vi "Test Serializer API.vi"() -> ()   [LabVIEW 2015, in "Serializer.lvlib"]
doc: "Serializer API Tester."
uses:
  Serializer.lvlib
panel:
  in  "close":bool
  in  "open":bool
  in  "conf":bool
  in  "config":string="{\"Plugin\":\"MOXAIP\",\"IP\":\"192.168.20.118\",\"Port\":4001}"
  in  "Send":bool
  in  "String":string
  in  "Run as Singleton?":bool
  in  "Show Block Diagram":bool
  in  "Refresh Modules":bool
  out "Active Modules":string[](array[string])
  in  "Stop Module":bool
  in  "Select Module":i32(ring)=-1 caption="Select Module\nTo send Request to" items=["All"=-1]
  in  "Run New Module":bool
  in  "Hide Module Panel":bool
  in  "Show Module Panel":bool
  out "Status":string
  # "This VI tests the API for the Module."
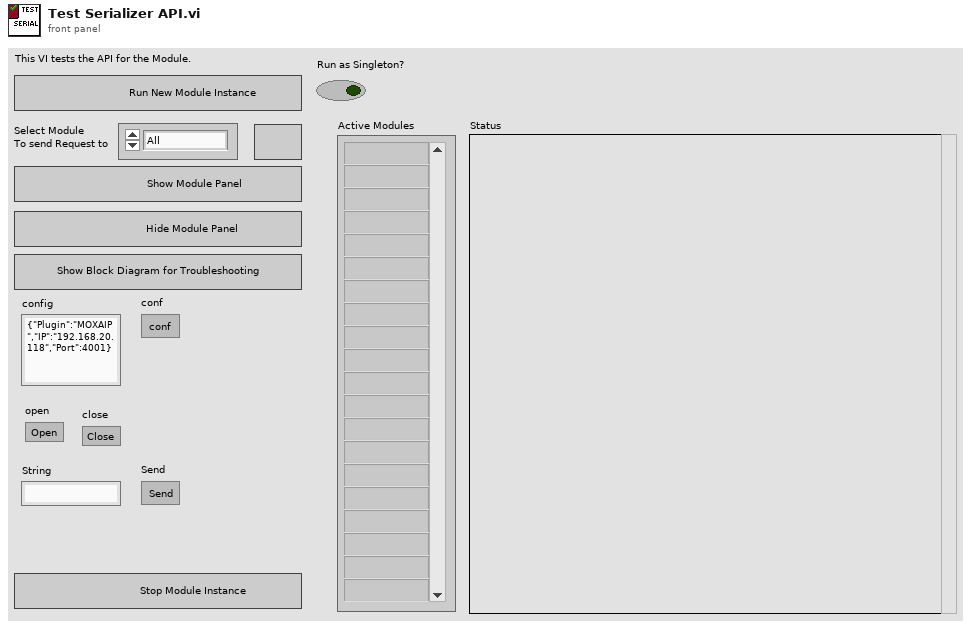
[diagram p1: front panel]
types:
  T1 = typedef "Serializer.lvlib/Broadcast Events--cluster.ctl" = cluster{"Module Did Init":refnum<user-event>, "Status Updated":refnum<user-event>, "Error Reported":refnum<user-event>, "Module Did Stop":refnum<user-event>, "Update Module Execution Status":refnum<user-event>, "Received":refnum<user-event>}
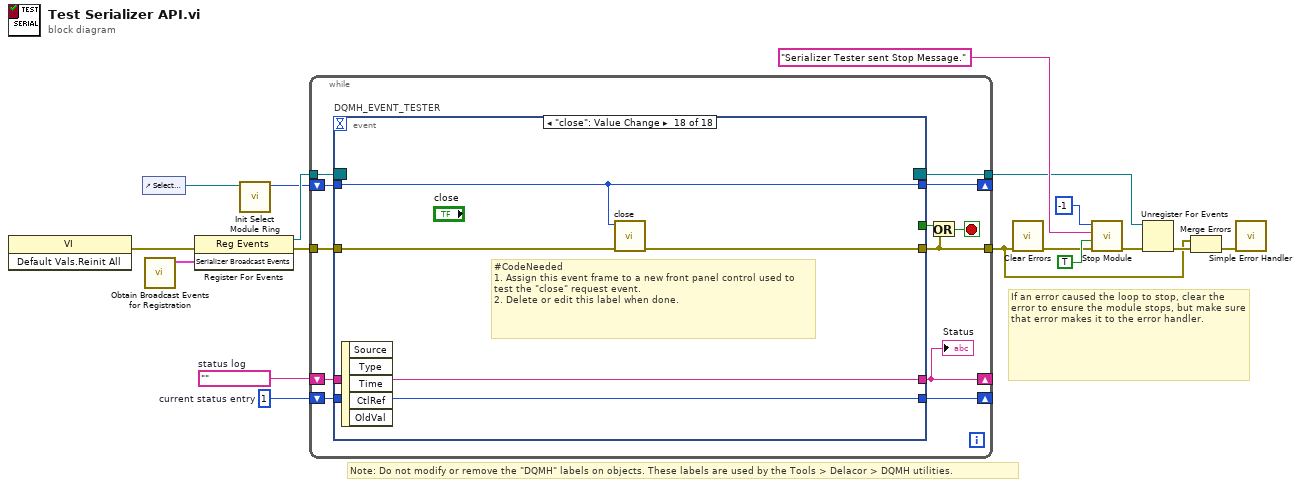
[diagram p0: block diagram]
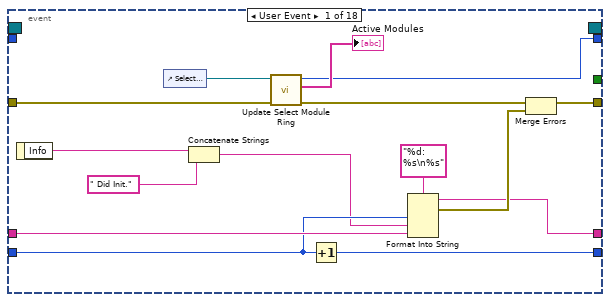
[diagram p2: hidden frame]
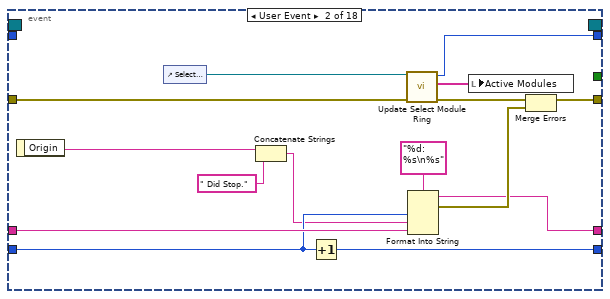
[diagram p3: hidden frame]
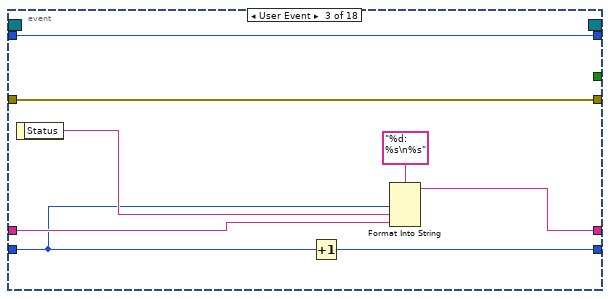
[diagram p4: hidden frame]
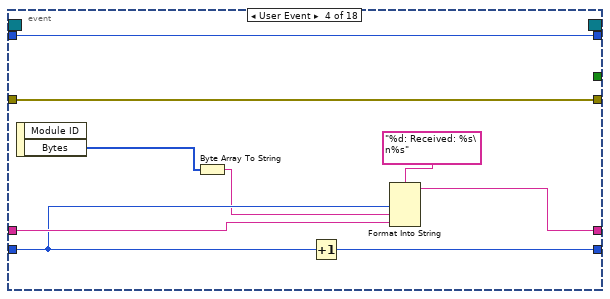
[diagram p5: hidden frame]
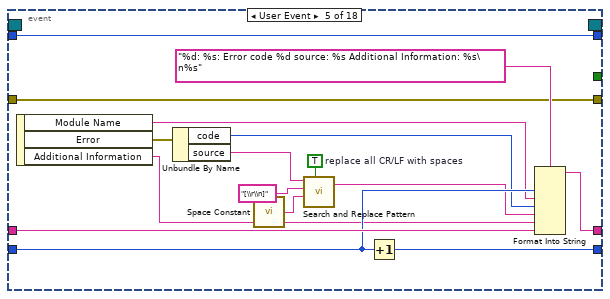
[diagram p6: hidden frame]
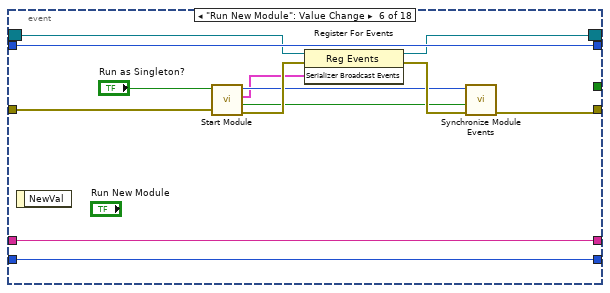
[diagram p7: hidden frame]
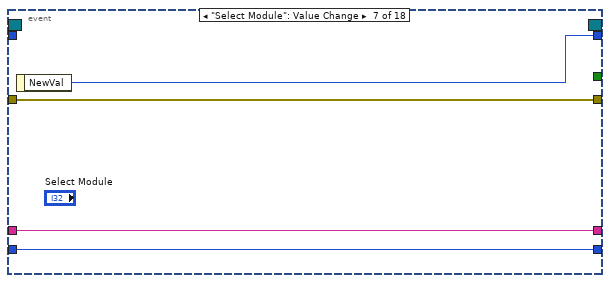
[diagram p8: hidden frame]
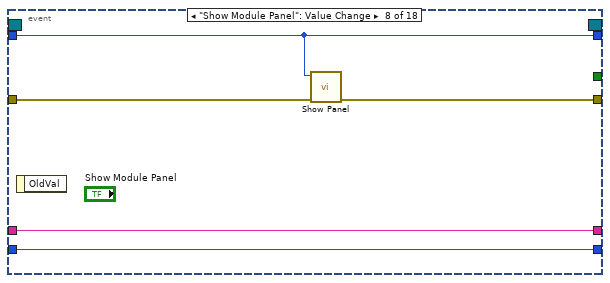
[diagram p9: hidden frame]
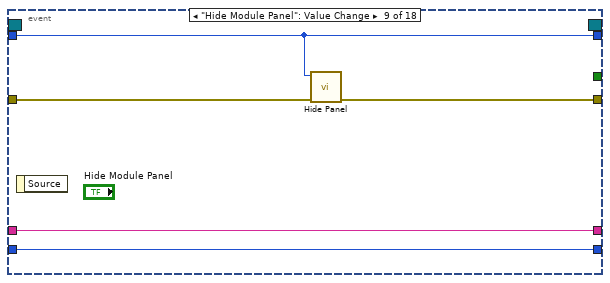
[diagram p10: hidden frame]
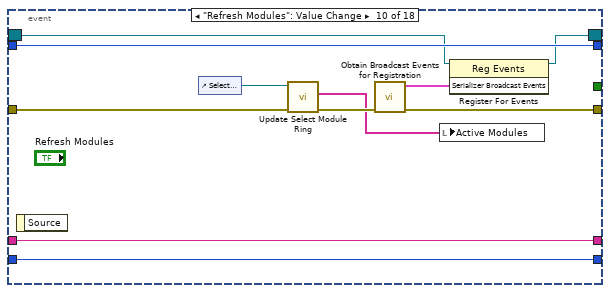
[diagram p11: hidden frame]
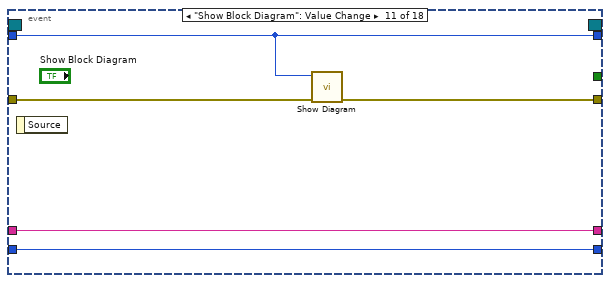
[diagram p12: hidden frame]
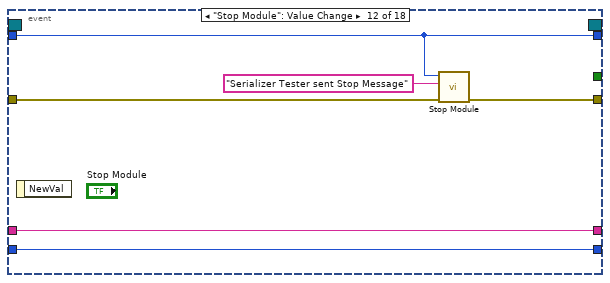
[diagram p13: hidden frame]
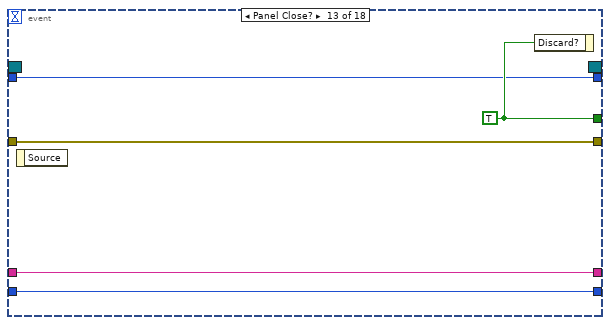
[diagram p14: hidden frame]
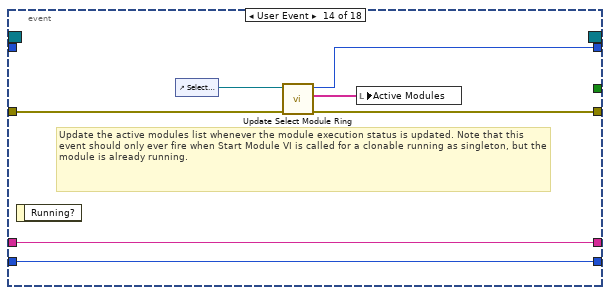
[diagram p15: hidden frame]
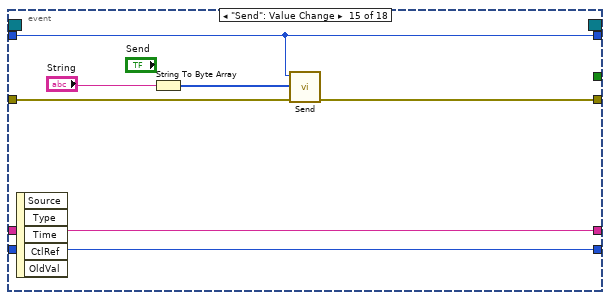
[diagram p16: hidden frame]
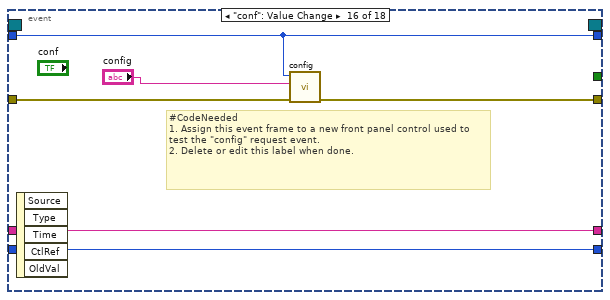
[diagram p17: hidden frame]
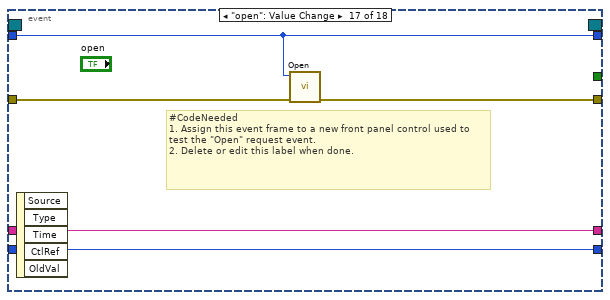
[diagram p18: hidden frame]
diagram:
  w13 = 1  # current status entry
  w14 = ""  # status log
  # "If an error caused the loop to stop, clear the error to ensure the module stops, but make sure that error makes it to the error handler."
  # "Note: Do not modify or remove the \"DQMH\" labels on objects. These labels are used by the Tools > Delacor > DQMH utilities."
  n1 = invoke class="VI" method="Default Vals.Reinit All"() -> (error out=w6:errorcluster)  [unwired: 3 in, 2 out]
  n2 = control-ref of="Select Module"() -> (w11:refnum<vi>)
  n3 = call "Obtain Broadcast Events for Registration.vi"() -> ("Serializer Broadcast Events"=w10:T1)  [unwired: 10 in, 1 out]
  n4 = register-events(error in=w6, w10) -> (reference out=w17:refnum<event-registration>, error out=w9:errorcluster)  [unwired: 1 in]
  n5 = call "Init Select Module Ring.vi"("Select Module Ring Ref"=w11) -> ("Value for All Modules"=w12:i32)  [unwired: 8 in, 2 out]
  n6 = while {
    tunnel: w17 -> [w29]
    tunnel: [w18] -> w1
    tunnel: w9 -> [w27]
    shift-right: [w23] -> _
    shift-left: w14 -> [w25]
    shift-right: [w24] -> _
    shift-left: w13 -> [w26]
    shift-right: [w20] -> _
    shift-left: w12 -> [w21]
    tunnel: [w19] -> w5
    stop <- w22 stop-if-true
    n7 = event "DQMH_EVENT_TESTER" shown="[17] \"close\": Value Change" {
      selector: w29 -> [_ _ _ _ _ w99 _ _ _ w125 _ _ _ _ _ _ _ _]
      dyn-events: [_ _ _ _ _ w98 _ _ _ w124 _ _ _ _ _ _ _ _] -> w19
      timeout: _ -> [_ _ _ _ _ _ _ _ _ _ _ _ _ _ _ _ _ _]
      tunnel: [_ _ _ _ _ _ _ _ _ _ _ _ w146 _ _ _ _ _] -> w28
      tunnel: [w33 w51 w67 w76 w82 w97 w109 w113 w118 w121 w132 w137 w145 w149 w157 w163 w168 w173] -> w18
      tunnel: w27 -> [w35 w53 w67 w76 w82 w100 w109 w114 w119 w126 w135 w138 w145 w150 w160 w166 w171 w176]
      tunnel: w26 -> [w41 w56 w60 w70 w88 w102 w107 w111 w116 w129 w133 w140 w143 w152 w158 w164 w169 w174]
      tunnel: w25 -> [w42 w57 w63 w72 w90 w103 w108 w112 w117 w130 w134 w141 w144 w153 w159 w165 w170 w175]
      tunnel: [w39 w54 w64 w73 w85 w103 w108 w112 w117 w130 w134 w141 w144 w153 w159 w165 w170 w175] -> w23
      tunnel: [w40 w55 w66 w75 w91 w102 w107 w111 w116 w129 w133 w140 w143 w152 w158 w164 w169 w174] -> w24
      tunnel: w21 -> [_ _ w61 w71 w92 w101 _ w110 w115 w128 w131 w139 w142 _ w156 w161 w167 w172]
      tunnel: [w30 w48 w61 w71 w92 w101 w106 w110 w115 w128 w131 w139 w142 w148 w156 w161 w167 w172] -> w20
      event User Event {
        n8 = event-data() -> ("Info"=w38:string)  [unwired: 1 in]
        n9 = control-ref of="Select Module"() -> (w32:refnum<vi>)
        n10 = Concatenate Strings(w38, " Did Init.") -> (w37:string)
        n11 = call "Update Select Module Ring.vi"("error in (no error)"=w35, "Select Module Ring Ref"=w32) -> ("error out"=w34:errorcluster, "Active Modules (Array)"=→"Active Modules":string[], "New Module Ring Value"=w30:i32)  [unwired: 7 in]
        n12 = Increment(x=w41) -> (x+1=w40:i32)
        n13 = Format Into String(format string="%d: %s\n%s", w41, w37, w42) -> (resulting string=w39:string, error out=w44:errorcluster)  [unwired: 2 in]
        n14 = Merge Errors(w34, w44) -> (w33:errorcluster)
      }
      event User Event {
        n15 = event-data() -> ("Origin"=w46:string)  [unwired: 1 in]
        n16 = control-ref of="Select Module"() -> (w50:refnum<vi>)
        n17 = Concatenate Strings(w46, " Did Stop.") -> (w45:string)
        n18 = Increment(x=w56) -> (x+1=w55:i32)
        n19 = call "Update Select Module Ring.vi"("error in (no error)"=w53, "Select Module Ring Ref"=w50) -> ("error out"=w52:errorcluster, "Active Modules (Array)"=w49:string[], "New Module Ring Value"=w48:i32)  [unwired: 7 in]
        n20 = Format Into String(format string="%d: %s\n%s", w56, w45, w57) -> (resulting string=w54:string, error out=w59:errorcluster)  [unwired: 2 in]
        n21 = local write "Active Modules"(w49) -> ()
        n22 = Merge Errors(w52, w59) -> (w51:errorcluster)
      }
      event User Event {
        n23 = event-data() -> ("Status"=w62:string)  [unwired: 1 in]
        n24 = Increment(x=w60) -> (x+1=w66:i32)
        n25 = Format Into String(format string="%d: %s\n%s", w60, w62, w63) -> (resulting string=w64:string)  [unwired: 2 in, 1 out]
      }
      event User Event {
        n26 = event-data() -> ("Bytes"=w69:u8[])  [unwired: 1 in, 1 out]
        n27 = Byte Array To String(unsigned byte array=w69) -> (string=w68:string)
        n28 = Increment(x=w70) -> (x+1=w75:i32)
        n29 = Format Into String(format string="%d: Received: %s\n%s", w70, w68, w72) -> (resulting string=w73:string)  [unwired: 2 in, 1 out]
      }
      event User Event {
        w86 = TRUE  # replace all CR/LF with spaces
        n30 = event-data() -> ("Module Name"=w80:string, "Error"=w79:errorcluster, "Additional Information"=w77:string)  [unwired: 1 in]
        n31 = Unbundle By Name(w79) -> ("code"=w81:i32, "source"=w83:string)
        n32 = call <vilib>:"Space Constant.vi"() -> ("String"=w87:string)
        n33 = call <vilib>:"Search and Replace Pattern.vi"("string"=w83, "regular expression (\"\")"="[\\r\\n]" ("regular expression (\"\")"), "replace string (\"\")"=w87, "replace all? (F)"=w86) -> ("result string"=w84:string)  [unwired: 1 in, 1 out]
        n34 = Increment(x=w88) -> (x+1=w91:i32)
        n35 = Format Into String(format string="%d: %s: Error code %d source: %s Additional Information: %s\n%s", w88, w80, w81, w84, w77, w90) -> (resulting string=w85:string)  [unwired: 2 in, 1 out]
      }
      event "Run New Module": Value Change {
        n36 = event-data() -> ()  [unwired: 1 in, 1 out]
        n37 = call "Start Module.vi"("error in (no error)"=w100, "Run as Singleton? (F)"="Run as Singleton?") -> ("error out"=w104:errorcluster, "Wait for Event Sync?"=w95:bool, "Serializer Broadcast Events"=w94:T1, "Module ID"=w96:i32)  [unwired: 6 in]
        n38 = register-events(reference=w99, error in=w104, w94) -> (reference out=w98:refnum<event-registration>, error out=w105:errorcluster)
        n39 = call "Synchronize Module Events.vi"("error in (no error)"=w105, "Wait for Event Sync?"=w95, "Module ID"=w96) -> ("error out"=w97:errorcluster)  [unwired: 7 in, 1 out]
      }
      event "Select Module": Value Change {
        n40 = event-data() -> ("NewVal"=w106:i32)  [unwired: 1 in]
      }
      event "Show Module Panel": Value Change {
        n41 = event-data() -> ()  [unwired: 1 in, 1 out]
        n42 = call "Show Panel.vi"("error in (no error)"=w114, "Module ID"=w110) -> ("error out"=w113:errorcluster)  [unwired: 9 in]
      }
      event "Hide Module Panel": Value Change {
        n43 = event-data() -> ()  [unwired: 1 in, 1 out]
        n44 = call "Hide Panel.vi"("error in (no error)"=w119, "Module ID"=w115) -> ("error out"=w118:errorcluster)  [unwired: 9 in]
      }
      event "Refresh Modules": Value Change {
        n45 = event-data() -> ()  [unwired: 1 in, 1 out]
        n46 = control-ref of="Select Module"() -> (w127:refnum<vi>)
        n47 = call "Update Select Module Ring.vi"("error in (no error)"=w126, "Select Module Ring Ref"=w127) -> ("error out"=w122:errorcluster, "Active Modules (Array)"=w120:string[])  [unwired: 7 in, 1 out]
        n48 = call "Obtain Broadcast Events for Registration.vi"("error in (no error)"=w122) -> ("error out"=w121:errorcluster, "Serializer Broadcast Events"=w123:T1)  [unwired: 9 in]
        n49 = local write "Active Modules"(w120) -> ()
        n50 = register-events(reference=w125, w123) -> (reference out=w124:refnum<event-registration>)  [unwired: 1 in, 1 out]
      }
      event "Show Block Diagram": Value Change {
        n51 = event-data() -> ()  [unwired: 1 in, 1 out]
        n52 = call "Show Diagram.vi"("error in (no error)"=w135, "Module ID"=w131) -> ("error out"=w132:errorcluster)  [unwired: 9 in]
      }
      event "Stop Module": Value Change {
        n53 = event-data() -> ()  [unwired: 1 in, 1 out]
        n54 = call "Stop Module.vi"("error in (no error)"=w138, "Origin"="Serializer Tester sent Stop Message", "Module ID"=w139) -> ("error out"=w137:errorcluster)  [unwired: 8 in]
      }
      event Panel Close? {
        w146 = TRUE ("Discard?")
        n55 = event-data() -> ()  [unwired: 1 in, 1 out]
        n56 = event-data("Discard?"=w146) -> ()  [unwired: 1 in, 1 out]
      }
      event User Event {
        # "Update the active modules list whenever the module execution status is updated. Note that this event should only ever fire when Start Module VI is called for a clonable running as singleton, but the module is already running."
        n57 = event-data() -> ()  [unwired: 1 in, 1 out]
        n58 = control-ref of="Select Module"() -> (w151:refnum<vi>)
        n59 = call "Update Select Module Ring.vi"("error in (no error)"=w150, "Select Module Ring Ref"=w151) -> ("error out"=w149:errorcluster, "Active Modules (Array)"=w147:string[], "New Module Ring Value"=w148:i32)  [unwired: 7 in]
        n60 = local write "Active Modules"(w147) -> ()
      }
      event "Send": Value Change {
        n61 = event-data() -> ()  [unwired: 1 in, 5 out]
        n62 = String To Byte Array(string="String") -> (unsigned byte array=w154:u8[])
        n63 = call "Send.vi"("error in (no error)"=w160, "Bytes"=w154, "Module ID"=w156) -> ("error out"=w157:errorcluster)  [unwired: 8 in]
      }
      event "conf": Value Change {
        # "#CodeNeeded\n1. Assign this event frame to a new front panel control used to test the \"config\" request event.\n2. Delete or edit this label when done."
        n64 = event-data() -> ()  [unwired: 1 in, 5 out]
        n65 = call "config.vi"("error in (no error)"=w166, "config"="config", "Module ID"=w161) -> ("error out"=w163:errorcluster)  [unwired: 8 in]
      }
      event "open": Value Change {
        # "#CodeNeeded\n1. Assign this event frame to a new front panel control used to test the \"Open\" request event.\n2. Delete or edit this label when done."
        n66 = event-data() -> ()  [unwired: 1 in, 5 out]
        n67 = call "Open.vi"("error in (no error)"=w171, "Module ID"=w167) -> ("error out"=w168:errorcluster)  [unwired: 9 in]
      }
      event "close": Value Change {
        # "#CodeNeeded\n1. Assign this event frame to a new front panel control used to test the \"close\" request event.\n2. Delete or edit this label when done."
        n68 = event-data() -> ()  [unwired: 1 in, 5 out]
        n69 = call "close.vi"("error in (no error)"=w176, "Module ID"=w172) -> ("error out"=w173:errorcluster)  [unwired: 9 in]
      }
    }
    "Status" <- w23
    n70 = Or(x=w28, y=w18) -> (x .or. y?=w22:bool)
  }
  n71 = call <vilib>:"Clear Errors.vi"("error in (no error)"=w1) -> ("error out"=w3:errorcluster)  [unwired: 5 in, 1 out]
  n72 = call "Stop Module.vi"("error in (no error)"=w3, "Wait for Module to stop? (F)"=TRUE ("Wait for Module to stop?"), "Origin"="Serializer Tester sent Stop Message.", "Module ID"=-1 ("Stop all")) -> ("error out"=w15:errorcluster)  [unwired: 7 in]
  n73 = Unregister For Events(event registration refnum=w5, error in=w15) -> (error out=w16:errorcluster)
  n74 = Merge Errors(w1, w16) -> (w2:errorcluster)
  n75 = call <vilib>:"Simple Error Handler.vi"("error in (no error)"=w2) -> ()  [unwired: 4 in, 5 out]
